vi "Array Manipulation.vi"() -> ()   [LabVIEW 2022 SP3]
doc: "This VI shows how different array functions can be used to manipulate data. There are also examples showing how we can use the Polymorphic functionality built into LabVIEW to easily modify the data in an array. \n\nExamine the different cases and read the comments on the block diagram for more details"
uses:
  <vilib>/measure/NI_MABase.lvlib
panel:
  in  "Stop Button":bool
  in  "Tab Control":T1(tab)
  out "Concatenated Data Array":dbl[](array[numeric])
  out "Concatenated Data":dbl[](graph)
  in  "Subtract?":bool
  out "Add or Subtract Data Array":dbl[](array[numeric])
  out "Add or Subtract Data":dbl[](graph)
  in  "Select Channel":u16(ring) items=["Channel 0", "Channel 1"]
  out "Single Channel of Data Array":dbl[](array[numeric])
  out "Single Channel of Data":dbl[](graph)
  out "Size of Array":i32
  in  "Offset":dbl(slide)=-8.326672684688674e-17 scale=-5.0..5.0
  out "Waveform Data":waveform(dbl)[](graph)
  out "Data Channel Array":dbl[][](array[numeric])
  in  "Channel 1 Offset":dbl(slide)=-8.326672684688674e-17 scale=-5.0..5.0
  out "All Data Channel":dbl[][](graph)
  out "Size of Array":i32[](array[numeric])
  out "Subset Data Array":dbl[][](array[numeric])
  in  "Start Value":i32(slide)=10 scale=0.0..1000.0
  out "Subset Data":dbl[][](graph)
  in  "Length":i32(slide)=1000 scale=0.0..1000.0
  # "Rows"
  # "Columns"
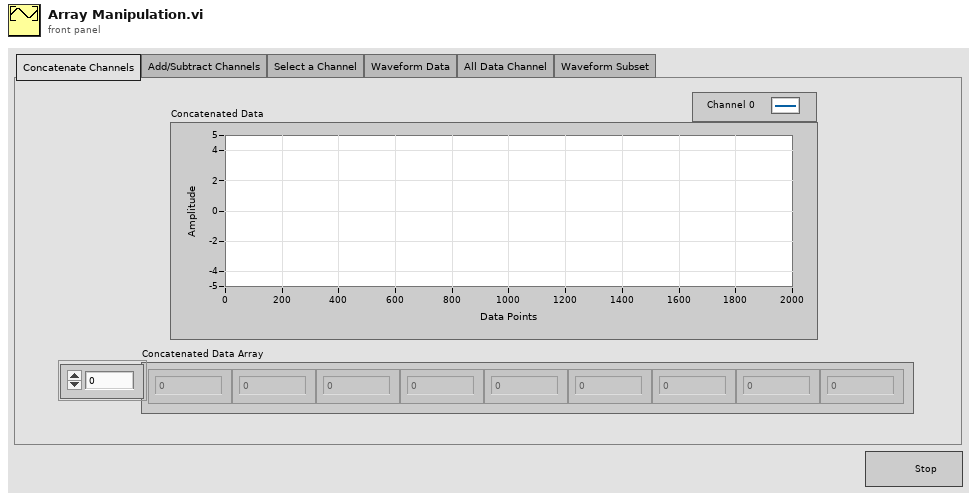
[diagram p1: front panel]
types:
  T1 = enum32{"Concatenate Channels", "Add/Subtract Channels", "Select a Channel", "Waveform Data", "All Data Channel", "Waveform Subset"}
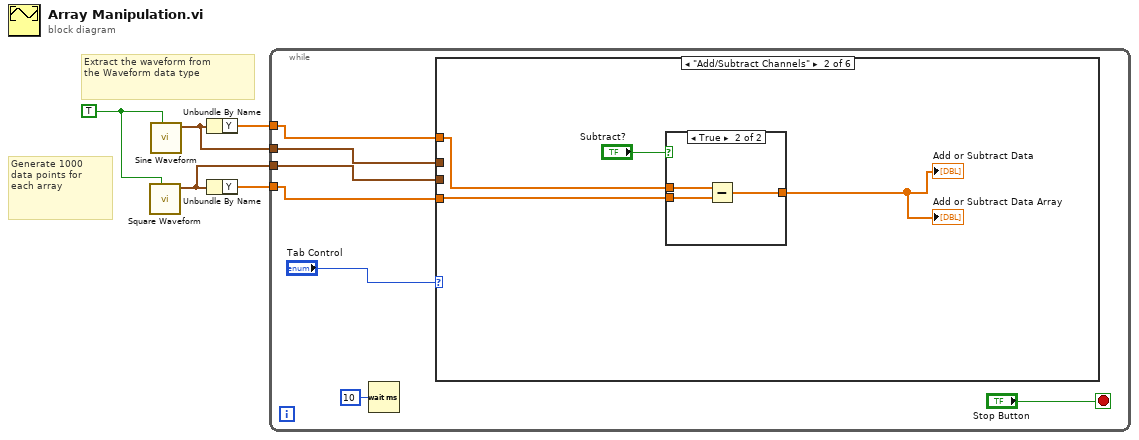
[diagram p0: block diagram]
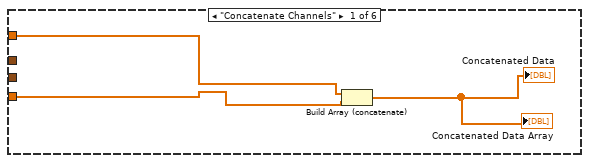
[diagram p2: hidden frame]
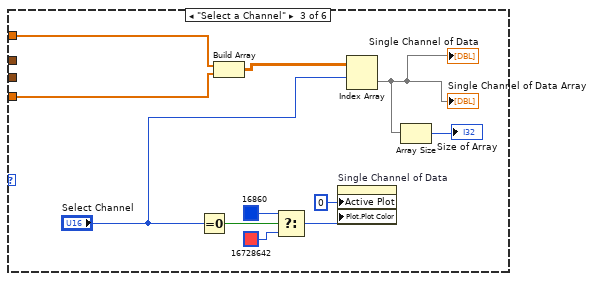
[diagram p4: hidden frame]
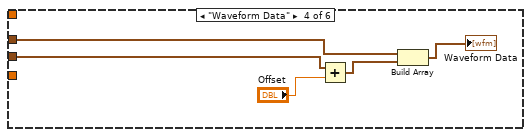
[diagram p5: hidden frame]
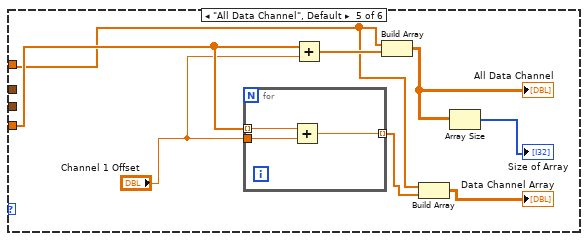
[diagram p6: hidden frame]
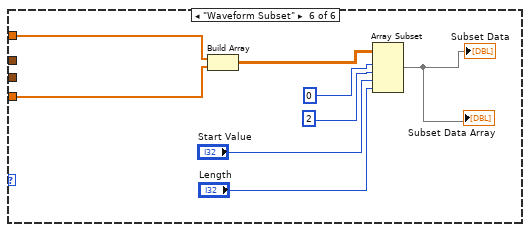
[diagram p7: hidden frame]
diagram:
  w5 = TRUE
  # "Extract the waveform from \nthe Waveform data type"
  # "Generate 1000\ndata points for \neach array"
  n1 = call <vilib>:"Square Waveform.vi"("reset signal"=w5) -> ("signal out"=w1:waveform(dbl))  [unwired: 9 in, 1 out]
  n2 = call <vilib>:"Sine Waveform.vi"("reset signal"=w5) -> ("signal out"=w2:waveform(dbl))  [unwired: 9 in, 1 out]
  n3 = Unbundle By Name(w2) -> ("Y"=w4:dbl[])
  n4 = Unbundle By Name(w1) -> ("Y"=w3:dbl[])
  n5 = while {
    tunnel: w4 -> [w7]
    tunnel: w3 -> [w6]
    tunnel: w2 -> [w10]
    tunnel: w1 -> [w9]
    stop <- "Stop Button" stop-if-true
    n6 = Wait (ms)(milliseconds to wait=u32 10) -> ()  [unwired: 1 out]
    n7 = case shown="\"Add/Subtract Channels\"" "Tab Control" {
      tunnel: w7 -> [w15 w17 w28 _ w43 w57]
      tunnel: w6 -> [w14 w18 w27 _ w46 w56]
      tunnel: w10 -> [_ _ _ w35 _ _]
      tunnel: w9 -> [_ _ _ w37 _ _]
      frame "Concatenate Channels" {
        n8 = Build Array (concatenate)(w15, w14) -> (→"Concatenated Data" →"Concatenated Data Array":dbl[])
      }
      frame "Add/Subtract Channels" {
        n9 = case shown="True" "Subtract?" {
          tunnel: w17 -> [_ w22]
          tunnel: w18 -> [_ w21]
          tunnel: [_ w20] -> w16
          frame False {
          }
          frame True {
            n10 = Subtract(x=w22, y=w21) -> (x-y=w20:dbl[])
          }
        }
        "Add or Subtract Data" <- w16
        "Add or Subtract Data Array" <- w16
      }
      frame "Select a Channel" {
        n11 = Equal To 0?(x="Select Channel") -> (x = 0?=w29:bool)
        n12 = Build Array(w28, w27) -> (w26:dbl[][])
        n13 = Select(t=u32 16860, s=w29, f=u32 16728642) -> (s? t:f=w32:u32)
        n14 = property on="Single Channel of Data" class="WFGraph (strict)"("Active Plot"=u32 0, "Plot.Plot Color"=w32) -> ()  [unwired: 2 in, 2 out]
        n15 = Index Array(array=w26, index (row)="Select Channel") -> (element=w23:dbl[])  [unwired: 1 in]
        "Single Channel of Data" <- w23
        "Single Channel of Data Array" <- w23
        n16 = Array Size(array=w23) -> (size(s)=→"Size of Array":i32)
      }
      frame "Waveform Data" {
        n17 = Add(x=w37, y="Offset") -> (x+y=w36:waveform(dbl))
        n18 = Build Array(w35, w36) -> (→"Waveform Data":waveform(dbl)[])
      }
      frame "All Data Channel", Default {
        n19 = for {
          tunnel: w46 -> [w49] mode=indexing
          tunnel: "Channel 1 Offset" -> [w48]
          tunnel: [w47] -> w42 mode=indexing
          n20 = Add(x=w49, y=w48) -> (x+y=w47:dbl)
        }
        n21 = Add(x=w46, y="Channel 1 Offset") -> (x+y=w44:dbl[])
        n22 = Build Array(w43, w44) -> (w40:dbl[][])
        "All Data Channel" <- w40
        n23 = Build Array(w43, w42) -> (→"Data Channel Array":dbl[][])
        n24 = Array Size(array=w40) -> (size(s)=→"Size of Array":i32[])
      }
      frame "Waveform Subset" {
        n25 = Build Array(w57, w56) -> (w55:dbl[][])
        n26 = Array Subset(array=w55, index (row)=0, length (row)=2, index (col)="Start Value", length (col)="Length") -> (→"Subset Data Array" →"Subset Data":dbl[][])
      }
    }
  }
